vi "Main FPGA.vi"(10 "Matrix Array":u8[](array[numeric])=[0, 0, 0, 0, 0, 0, 0, 0, 0, 0, 0, 0, 0, 0, 0, 0, 0, 0, 0, 0, 0, 0, 0, 0, 0, 0, 0, 0, 0, 0, 0, 0, 0, 0, 0, 0, 0, 0, 0, 0, 0, 0, 0, 0, 0, 0, 0, 0, 0, 0, 0, 0, 0, 0, 0, 0, 0, 0, 0, 0, 0, 0, 0, 0, 0, 0, 0, 0, 0, 0, 0, 0, 0, 0, 0, 0, 0, 0, 0, 0, 0, 0, 0, 0, 0, 0, 0, 0, 0, 0, 0, 0, 0, 0, 0, 0, 0, 0, 0, 0, 0, 0, 0, 0, 0, 0, 0, 0, 0, 0, 0, 0, 0, 0, 0, 0, 0, 0, 0, 0, 0, 0, 0, 0, 0, 0, 0, 0, 0, 0, 0, 0, 0, 0, 0, 0, 0, 0, 0, 0, 0, 0, 0, 0, 0, 0, 0, 0, 0, 0, 0, 0, 0, 0, 0, 0, 0, 0, 0, 0, 0, 0, 0, 0, 0, 0, 0, 0, 0, 0, 0, 0, 0, 0, 0, 0, 0, 0, 0, 0, 0, 0, 0, 0, 0, 0, 0, 0, 0, 0, 0, 0], 11 "Update":bool) -> (3 "Timed Out?":bool)   [LabVIEW 2019]
uses:
  <vilib>/Platform/TimedLoop/XDataNode/timing_clust.ctl
  <vilib>/Platform/TimedLoop/XDataNode/nitl_modes.ctl
  <vilib>/Platform/TimedLoop/XDataNode/wakeup.ctl
  <vilib>/rvi/Emulation/niFpgaGetClockAttributes.vi
  <vilib>/rvi/Emulation/niFpgaSctlEmulationGetInTimedLoop.vi
  <vilib>/rvi/Emulation/niFpgaEmulationReportErrorSimple.vi
  <vilib>/rvi/Memory/Memory_Emulation/nirvimemoryFastEmulation.vi
  <vilib>/rvi/Memory/Memory_Emulation/nirvimemoryEmulation.vi
  <vilib>/rvi/Emulation/niFpgaEmulationIsFPGAContextNoSignature.vi
  <vilib>/rvi/DataTransferAndStorage/Container/Common/niFpgaContainerGetUniqueNameForEmu.vi
  <vilib>/rvi/Emulation/niFpgaProcessEmulError.vi
  <vilib>/rvi/errors/nirviReportUnexpectedCaseInternalError (U32).vi
  <vilib>/rvi/Emulation/niFpgaCriticalErrorInLSC.vi
  <vilib>/rvi/eio/common/nirviEmuTemplateMethod_errors.vi
  <vilib>/rvi/interface/RandomDataEmulation/niFpgaRandomDataHandleErrors.vi
  <vilib>/rvi/DataTransferAndStorage/Container/XNode/niFpgaContainer.xnode
  <vilib>/eio/EIONode/EIONode.xnode
  <vilib>/Platform/TimedLoop/XDataNode/XDataNode.xnode
  <vilib>/rvi/interface/RandomDataEmulation/nirviRandomDataFpgaReadWriteTemplate.vi
  <vilib>/Platform/TimedLoop/XDataNode/XDNodeRunTimeDep.lvlib
panel:
  in  "Reset (us)":u16=310
  in  "Low False":u8=34
  in  "Low True":u8=18
  in  "High False":u8=16
  in  "High True":u8=32
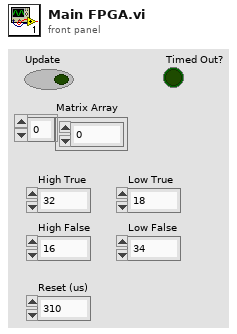
[diagram p1: front panel]
types:
  T1 = typedef "XDNodeRunTimeDep.lvlib/timing_clust.ctl" = cluster{"Expected End [f-1]":u64, "Actual End [f-1]":u64, "Finished Late? [f-1]":bool, "Expected End [i-1]":u64, "Actual End [i-1]":u64, "Finished Late? [i-1]":bool, "Expected Start [i]":u64, "Actual Start [i]":u64, "Expected Start [f]":u64, "Actual Start [f]":u64, "Source Name":string, "Structure Name":string, "Period":i64, "Deadline":i64, "Offset":i64, "Start":i64, "Priority":i32, "Timeout":i32, "Mode":T2, "Wakeup Reason":T3, "Error":errorcluster, "Source Type":string, "Secondary Source Type":string, "Global End Time":u64, "Global Start Time":u64, "Frame Duration":u64, "Iteration Duration":u64, "Assigned CPU":i32, "I/O Scan Engine Mode":u32}
  T2 = typedef "XDNodeRunTimeDep.lvlib/nitl_modes.ctl" = enum32{"No Change", "Process missed periods, maintain original phase", "Discard missed periods, maintain original phase", "Process missed periods, ignore original phase", "Discard missed periods, ignore original phase"}
  T3 = typedef "XDNodeRunTimeDep.lvlib/wakeup.ctl" = enum32{"Normal", "Aborted", "Asynchronous wakeup", "Timing source error", "Timed loop error", "Timeout"}
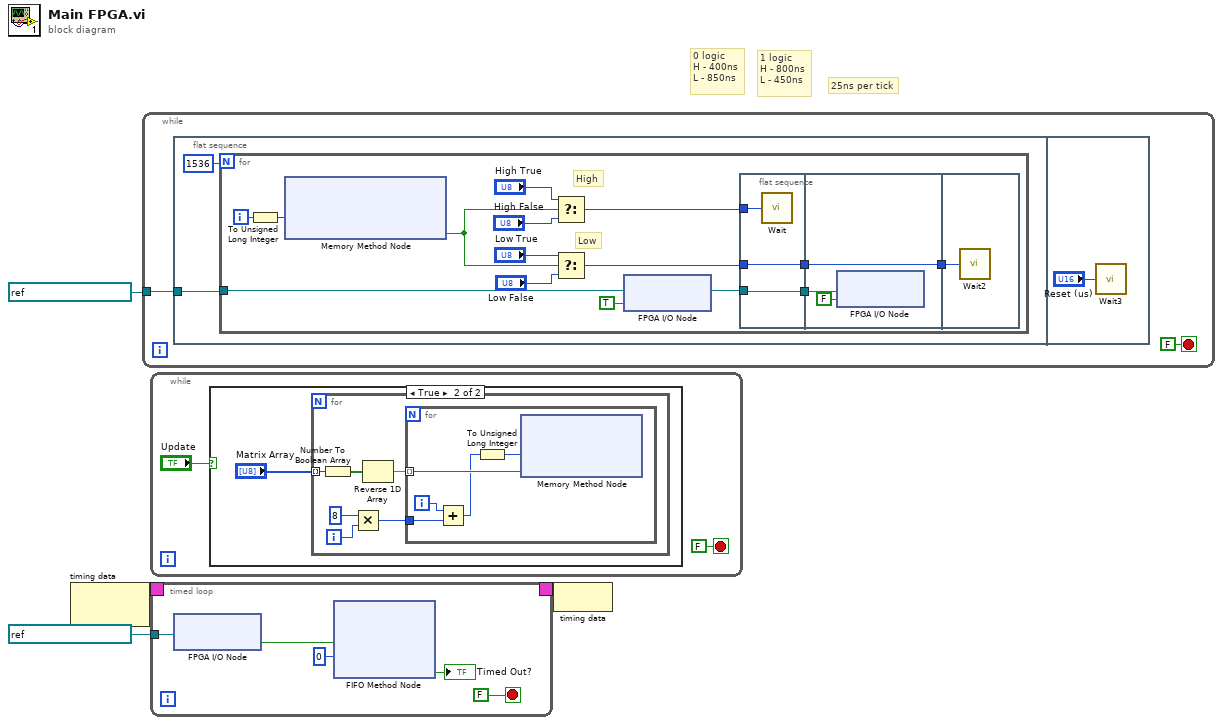
[diagram p0: block diagram]
diagram:
  # "1 logic\nH - 800ns\nL - 450ns"
  # "0 logic\nH - 400ns\nL - 850ns"
  # "25ns per tick"
  n1 = node-c288() -> (w2:T1)  [unwired: 1 in]
  n2 = while {
    tunnel: refnum<k21> "ConnectorC/DIO0" ("FPGA I/O In") -> [w5]
    stop <- FALSE stop-if-true
    n3 = flat-sequence {
      tunnel: w5 -> [w8]
      frame #0 {
        n4 = for {
          N: 1536 -> [_]
          tunnel: w8 -> [w10]
          i -> [w22]
          # "Low"
          # "High"
          n5 = To Unsigned Long Integer(number=w22) -> (unsigned 32bit integer=w23:u32)
          n6 = xnode ("Memory Method Node")("Address"=w23) -> ("Data"=w15:bool)  [unwired: 1 in, 1 out]
          n7 = Select(t="High True", s=w15, f="High False") -> (s? t:f=w20:u8)
          n8 = Select(t="Low True", s=w15, f="Low False") -> (s? t:f=w14:u8)
          n9 = xnode "FPGA I/O Node"("I/O Item"=TRUE, "FPGA I/O In"=w10) -> ("FPGA I/O Out"=w9:refnum<k21>)
          n10 = flat-sequence {
            tunnel: [w25] -> w21
            tunnel: [w26] -> w12
            tunnel: w14 -> [w26]
            tunnel: w20 -> [w24]
            tunnel: w9 -> [w25]
            tunnel: w21 -> [w29]
            tunnel: [w27] -> w13
            tunnel: w12 -> [w27]
            tunnel: w13 -> [w30]
            frame #0 {
              n11 = call "Wait"("Count(Ticks)"=w24) -> ()  [unwired: 1 out]
            }
            frame #1 {
              n12 = xnode "FPGA I/O Node"("I/O Item"=FALSE, "FPGA I/O In"=w29) -> ()  [unwired: 1 out]
            }
            frame #2 {
              n13 = call "Wait2"("Count(Ticks)"=w30) -> ()  [unwired: 1 out]
            }
          }
        }
      }
      frame #1 {
        n14 = call "Wait3"("Count(uSec)"="Reset (us)") -> ()  [unwired: 1 out]
      }
    }
  }
  n15 = while {
    stop <- FALSE stop-if-true
    n16 = case shown="True" "Update" {
      frame False {
      }
      frame True {
        n17 = for {
          tunnel: "Matrix Array" -> [w37] mode=indexing
          i -> [w40]
          n18 = Number To Boolean Array(number=w37) -> (Boolean array=w36:bool[])
          n19 = Multiply(x=8, y=w40) -> (x*y=w38:i32)
          n20 = Reverse 1D Array(array=w36) -> (reversed array=w35:bool[])
          n21 = for {
            tunnel: w35 -> [w44] mode=indexing
            tunnel: w38 -> [w42]
            i -> [w43]
            n22 = Add(x=w43, y=w42) -> (x+y=w41:i32)
            n23 = To Unsigned Long Integer(number=w41) -> (unsigned 32bit integer=w45:u32)
            n24 = xnode ("Memory Method Node")("Address"=w45, "Data"=w44) -> ()  [unwired: 1 in, 1 out]
          }
        }
      }
    }
  }
  n25 = timed-loop {
    tunnel: refnum<k21> "ConnectorC/DIO1" ("FPGA I/O In") -> [w50]
    timing: w2 -> [_]
    timing-out: [_] -> w1
    stop <- FALSE stop-if-true
    n26 = xnode "FPGA I/O Node"("FPGA I/O In"=w50) -> ("I/O Item"=w48:bool)  [unwired: 1 out]
    n27 = xnode ("FIFO Method Node")("Element"=w48, "Timeout"=0 ("Count(Ticks)")) -> ("Timed Out?"=→"Timed Out?":bool)  [unwired: 1 in, 1 out]
  }
  n28 = node-c288(w1) -> ()
